vi "WrtID.vi"(10 "id":u32, 11 "element in":T1) -> (3 "element out":T1)   [LabVIEW 2019, in "MessengerM.lvlib" / "SubChannelCPU.lvclass"]
uses:
  SubChannelCPU.lvclass
  <vilib>/ChannelSupport/Channel Message/Channel Message.lvclass
  Element.ctl
  MessengerM.lvlib
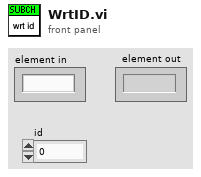
[diagram p1: front panel]
types:
  T1 = typedef "MessengerM.lvlib/Element.ctl" = string
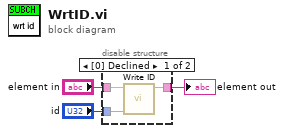
[diagram p0: block diagram]
diagram:
  n1 = disable-structure shown="[0] Declined" {
    disable-tunnel: "element in" -> [w6 w7]
    disable-tunnel: [w5 w7] -> w2
    disable-tunnel: "id" -> [w4 _]
    frame Disabled {
      n2 = call <vilib>:"Write ID.vi"("id"=w4, "Channel Message in"=w6) -> ("Channel Message out"=w5:refnum<class "Channel Message.lvclass">)  [unwired: 9 in]
    }
    frame Enabled {
    }
  }
  "element out" <- w2
